vi "SumOfFactorials.vi"() -> ()   [LabVIEW 2020]
panel:
  in  "Stop":bool
  out "Sum Of Factorial":i32
  in  "N":i32
  # "Sum of Factorials"
  # "This vi helps to find the sum of\nfactorial of the whole number"
  # "This is to stop the conversion process\nonce the vi is started."
  # "Working:\n1. The whole number should be given as the input.\n2. Then the sum will be shown in sum of  Factorial indicator"
  # "Disclaimer:\nThis vi will work only for output less than 2,147,483,647. Other than this value will result in error."
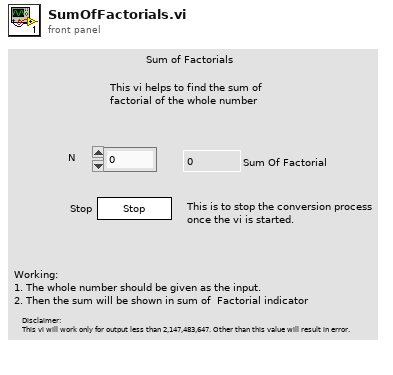
[diagram p1: front panel]
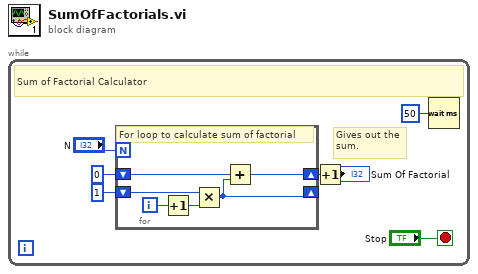
[diagram p0: block diagram]
diagram:
  n1 = while {
    stop <- "Stop" stop-if-true
    # "Gives out the\nsum."
    # "Sum of Factorial Calculator"
    n2 = for {
      N: "N" -> [_]
      shift-right: [w11] -> w4
      shift-left: 0 -> [w12]
      shift-right: [w10] -> _
      shift-left: 1 -> [w13]
      i -> [w9]
      # "For loop to calculate sum of factorial"
      n3 = Increment(x=w9) -> (x+1=w8:i32)
      n4 = Multiply(x=w13, y=w8) -> (x*y=w10:i32)
      n5 = Add(x=w12, y=w10) -> (x+y=w11:i32)
    }
    n6 = Increment(x=w4) -> (x+1=→"Sum Of Factorial":i32)
    n7 = Wait (ms)(milliseconds to wait=u32 50) -> ()  [unwired: 1 out]
  }
